vi "Serial_Arduino_LED.vi"() -> ()   [LabVIEW 2018]
uses:
  <vilib>/Instr/_visa.llb/VISA Configure Serial Port (Instr).vi
panel:
  out "write buffer":string
  in  "stop":bool
  in  "VISA resource name":refnum<visa-resource-name>
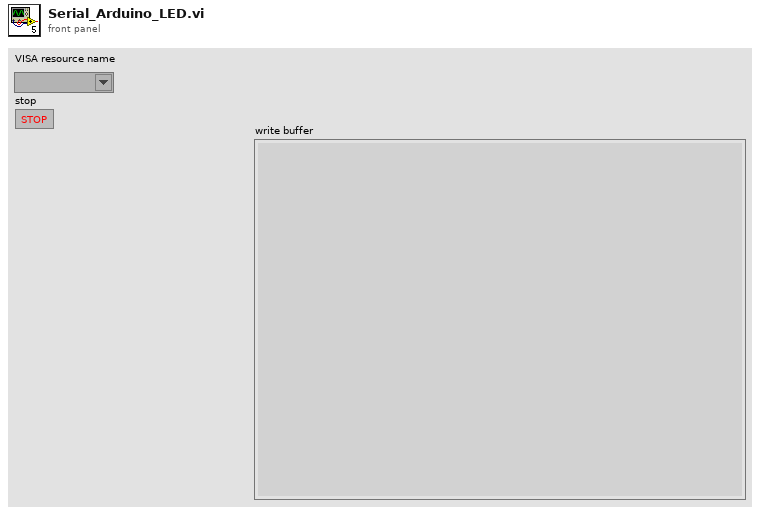
[diagram p1: front panel]
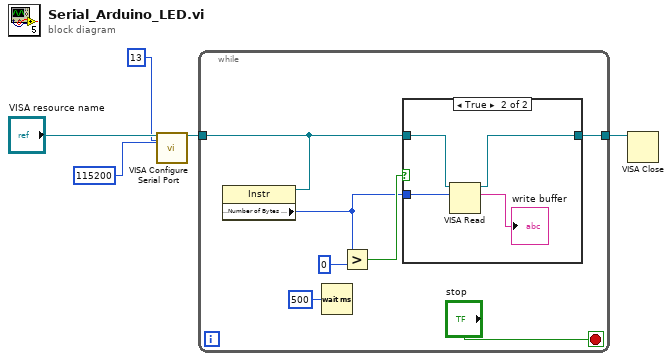
[diagram p0: block diagram]
diagram:
  n1 = call-poly "VISA Configure Serial Port"("VISA resource name"="VISA resource name", "termination char\n(0xA = '\\n' = LF)"=u8 13 ("termination char\n(0xA = '\\n' = LF)"), "baud rate (9600)"=u32 115200) -> ("VISA resource name out"=w4:refnum<visa-resource-name>)  [unwired: 11 in, 1 out]
  n2 = while {
    tunnel: w4 -> [w10]
    tunnel: [w11] -> w1
    stop <- "stop" stop-if-true
    n3 = property class="Instr"(reference=w10) -> ("Serial Settings:Number of Bytes at Serial Port"=w7:u32)  [unwired: 1 in, 2 out]
    n4 = Wait (ms)(milliseconds to wait=u32 500) -> ()  [unwired: 1 out]
    n5 = Greater?(x=w7, y=u32 0) -> (0:w9:bool)
    n6 = case shown="True" w9 {
      tunnel: [w13 w16] -> w11
      tunnel: w10 -> [w13 w15]
      tunnel: w7 -> [_ w14]
      frame False {
      }
      frame True {
        n7 = VISA Read(VISA resource name=w15, byte count=w14) -> (VISA resource name out=w16:refnum<visa-resource-name>, read buffer=→"write buffer":string)  [unwired: 1 in, 2 out]
      }
    }
  }
  n8 = VISA Close(VISA resource name=w1) -> ()  [unwired: 1 in, 1 out]
